vi "GSCalculation.vi"(0 "[d24]":dbl, 4 "[d13]":dbl=1.0, 5 "[O_B]":dbl=11.392382945373926, 6 "V_DC":dbl[][](array[numeric]), 7 "[M/B]":dbl, 8 "V_IF (1.5pi)":dbl[][](array[numeric]), 9 "V_IF (pi)":dbl[][](array[numeric]), 10 "V_IF (0.5pi)":dbl[][](array[numeric]), 11 "V_IF (0)":dbl[][](array[numeric])) -> (2 "S":dbl[][](array[numeric]), 3 "G":dbl[][](array[numeric]))   [LabVIEW 2015]
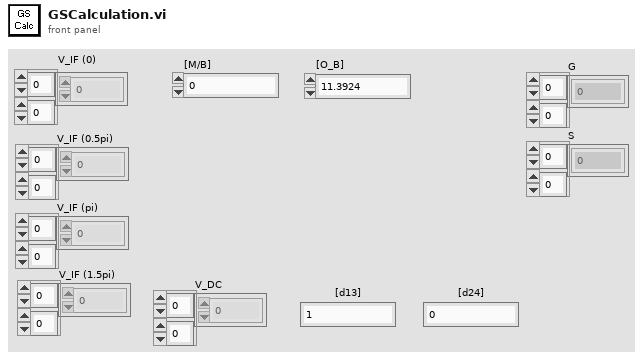
[diagram p1: front panel]
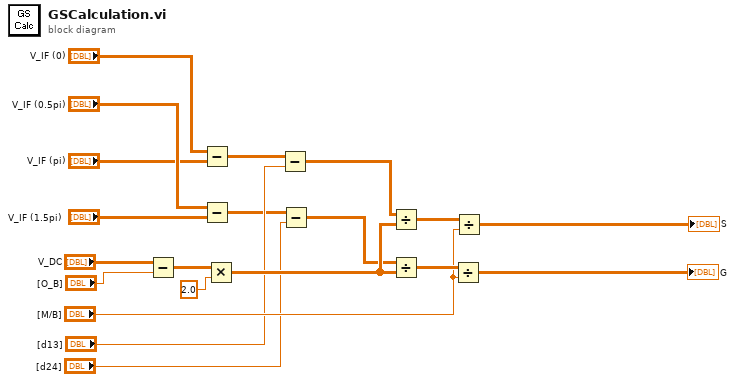
[diagram p0: block diagram]
diagram:
  n1 = Subtract(x="V_DC", y="[O_B]") -> (x-y=w11:dbl[][])
  n2 = Subtract(x="V_IF (0)", y="V_IF (pi)") -> (x-y=w6:dbl[][])
  n3 = Subtract(x="V_IF (0.5pi)", y="V_IF (1.5pi)") -> (x-y=w3:dbl[][])
  n4 = Multiply(x=w11, y=2.0 ("[O_B]")) -> (x*y=w10:dbl[][])
  n5 = Subtract(x=w6, y="[d13]") -> (x-y=w5:dbl[][])
  n6 = Subtract(x=w3, y="[d24]") -> (x-y=w2:dbl[][])
  n7 = Divide(x=w5, y=w10) -> (x/y=w16:dbl[][])
  n8 = Divide(x=w2, y=w10) -> (x/y=w15:dbl[][])
  n9 = Divide(x=w15, y="[M/B]") -> (x/y=→"G":dbl[][])
  n10 = Divide(x=w16, y="[M/B]") -> (x/y=→"S":dbl[][])
